vi "CMD_StoreBlueToothAddress.vi"(0 "Input_Data":string[](array[string]), 5 "Error In":errorcluster) -> (12 "Validate CheckSum":bool, 13 "Command":u8[](array[numeric])=[5, 247, 4, 128, 255, 0, 0, 0, 0, 0, 0, 0, 0, 0] format="%x", 14 "Response":bool, 15 "Ack":bool, 16 "Command":bool, 17 "Add CheckSum":bool, 18 "Status":bool, 19 "Error Out":errorcluster)   [LabVIEW 2014]
panel:
  # "Flags"
  # "Store BT Address Command:"
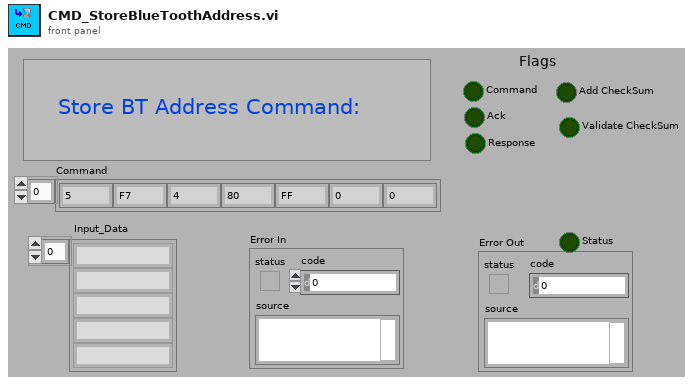
[diagram p1: front panel]
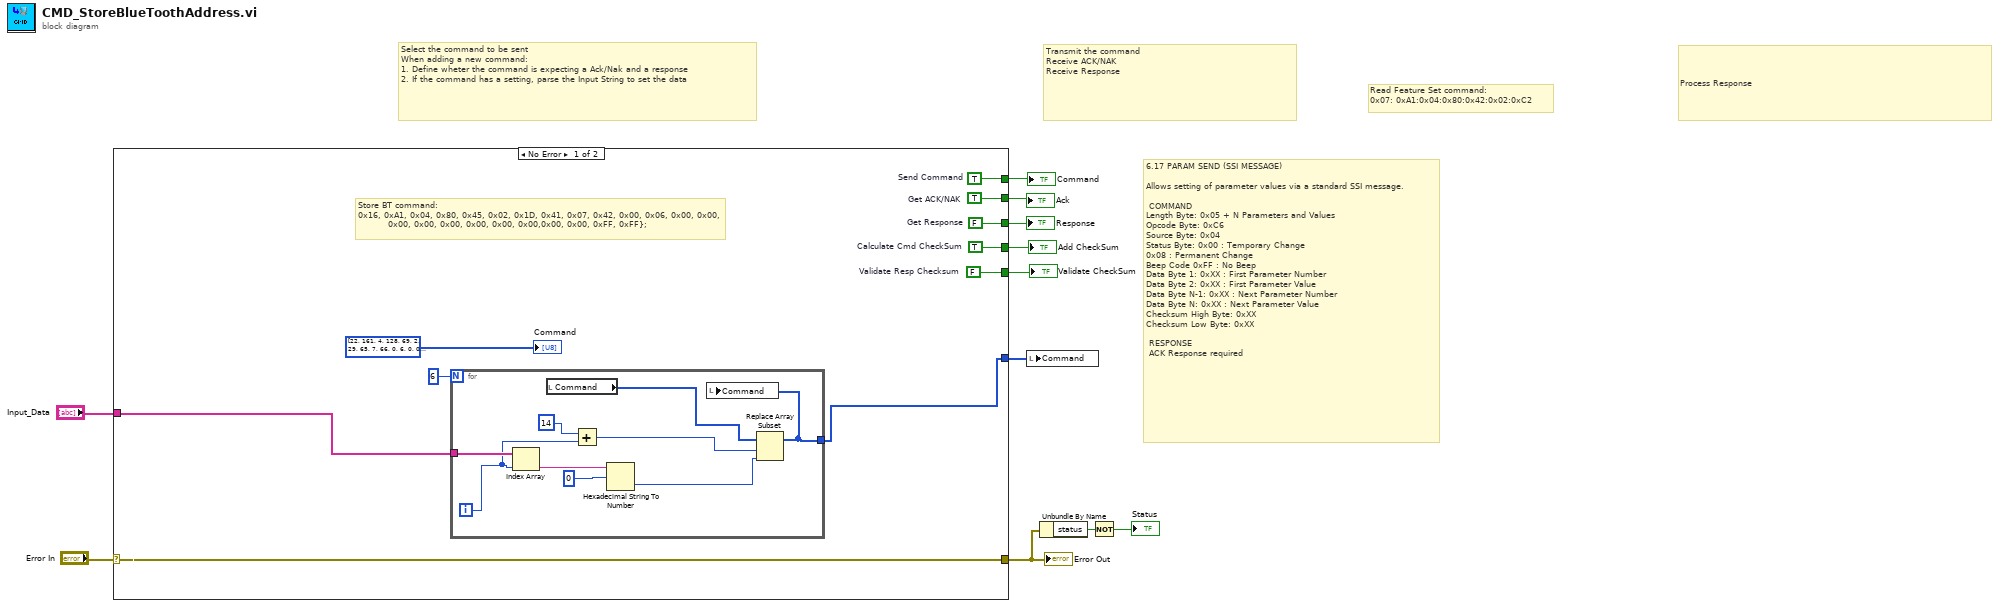
[diagram p0: block diagram]
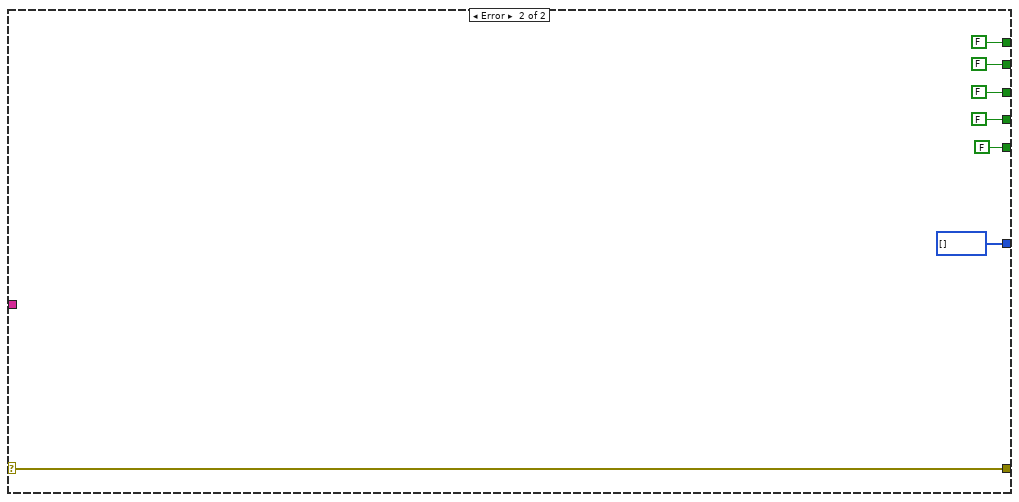
[diagram p2: hidden frame]
diagram:
  # "6.17\tPARAM SEND (SSI MESSAGE)\n\nAllows setting of parameter values via a standard SSI message.\n\n\tCOMMAND\nLength Byte:\t0x05 + N Parameters and Values\nOpcode Byte:\t0xC6\nSource Byte:\t0x04\nStatus Byte:\t0x00 : Temporary Change\n0x08 : Permanent Change\nBeep Code\t0xFF : No Beep\nData Byte 1:\t0xXX : First Parameter Number\nData Byte 2:\t0xXX : First Parameter Value\nData Byte N-1:\t0xXX : Next Parameter Number\nData Byte N:\t0xXX : Next Parameter Value\nChecksum High Byte:\t0xXX\nChecksum Low Byte:\t0xXX\n\n\tRESPONSE\n\tACK Response required"
  # "Read Feature Set command:\n0x07: 0xA1:0x04:0x80:0x42:0x02:0xC2"
  # "Process Response"
  # "Transmit the command\nReceive ACK/NAK\nReceive Response"
  # "Select the command to be sent\nWhen adding a new command:\n1. Define wheter the command is expecting a Ack/Nak and a response\n2. If the command has a setting, parse the Input String to set the data"
  n1 = case shown="No Error" "Error In" {
    selector: "Error In" -> [w17 w32]
    tunnel: [w21 FALSE ("Send Command")] -> w10
    tunnel: [w20 FALSE ("Get ACK/NAK")] -> w9
    tunnel: [w19 FALSE ("Get Response")] -> w8
    tunnel: [w18 FALSE ("Add CheckSum")] -> w7
    tunnel: [w13 u8[] []] -> w1
    tunnel: [w17 w32] -> w5
    tunnel: "Input_Data" -> [w14 _]
    tunnel: [w16 FALSE ("Validate Resp Checksum")] -> w2
    frame No Error {
      w16 = FALSE  # Validate Resp Checksum
      w18 = TRUE  # Calculate Cmd CheckSum
      w19 = FALSE  # Get Response
      w21 = TRUE  # Send Command
      w20 = TRUE  # Get ACK/NAK
      # "Store BT command:\n0x16, 0xA1, 0x04, 0x80, 0x45, 0x02, 0x1D, 0x41, 0x07, 0x42, 0x00, 0x06, 0x00, 0x00, \n\t\t\t\t\t\t\t\t\t\t0x00, 0x00, 0x00, 0x00, 0x00, 0x00,0x00, 0x00, 0xFF, 0xFF};"
      n2 = for {
        N: 6 -> [_]
        tunnel: w14 -> [w30]
        tunnel: [w22] -> w13
        i -> [w27]
        n3 = Index Array(array=w30, index=w27) -> (element=w26:string)
        n4 = local read "Command"() -> (w23:u8[])
        n5 = Add(x=14 ("index"), y=w27) -> (x+y=w28:i32)
        n6 = Hexadecimal String To Number(string=w26, offset=0) -> (number=w24:u32)  [unwired: 1 in, 1 out]
        n7 = Replace Array Subset(array=w23, new element=w24, index=w28) -> (w22:u8[])
        n8 = local write "Command"(w22) -> ()
      }
      "Command" <- u8[] [22, 161, 4, 128, 69, 2, 29, 65, 7, 66, 0, 6, 0, 0, 0, 0, 0, 0, 0, 0, 255, 255, 255, 0, 0, 0]
    }
    frame Error {
    }
  }
  "Error Out" <- w5
  "Command" <- w10
  "Ack" <- w9
  "Response" <- w8
  "Add CheckSum" <- w7
  "Validate CheckSum" <- w2
  n9 = local write "Command"(w1) -> ()
  n10 = Unbundle By Name(w5) -> ("status"=w4:bool)
  n11 = Not(x=w4) -> (.not. x?=→"Status":bool)
